vi "Set measurement.vi"(8 "error in (no error)":errorcluster, 10 "Measurement settings":T1={"Source Mode "=0, "Source Level"=0.0, "Source Limit"=0.0, "Measure Function"=1, "Remote sense"=FALSE, "Clear buffer?"=FALSE, "Beep"=FALSE, "High Capacity"=FALSE, "Terminals"=0, "PLCs"=1.0, "Fast measurement"=FALSE} {"Measure Function" items=["Volts", "Current", "Auto Resistance", "Manual Resistance", "Digitize Voltage", "Digitize Current"]; "Source Mode" items=["Voltage", "Current"]; "Terminals" items=["Front", "Rear"]}, 11 "SMU status in":T2 {"Measure Function" items=["Volts", "Current", "Auto Resistance", "Manual Resistance", "Digitize Voltage", "Digitize Current"]; "Source Mode" items=["Voltage", "Current"]}) -> (0 "error out":errorcluster, 3 "SMU status out":T2 {"Measure Function" items=["Volts", "Current", "Auto Resistance", "Manual Resistance", "Digitize Voltage", "Digitize Current"]; "Source Mode" items=["Voltage", "Current"]})   [LabVIEW 2017]
uses:
  ctls/SMU status.ctl
  ctls/SMU settings.ctl
  <instrlib>/Keithley 2450/Keithley 2450.lvlib
  Source meter.lvlib
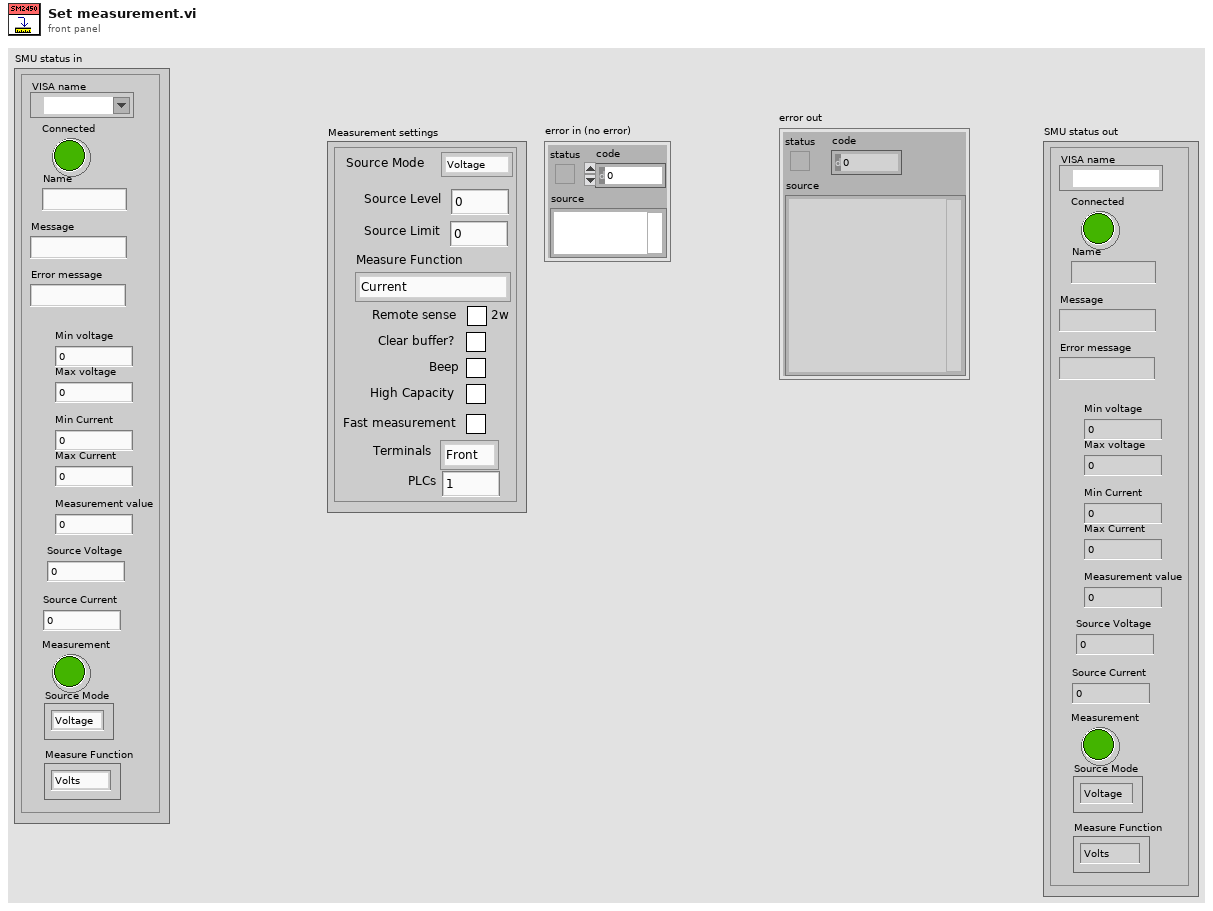
[diagram p1: front panel]
types:
  T1 = typedef "SMU settings.ctl" = cluster{"Source Mode ":u16, "Source Level":dbl, "Source Limit":dbl, "Measure Function":u16, "Remote sense":bool, "Clear buffer?":bool, "Beep":bool, "High Capacity":bool, "Terminals":u16, "PLCs":dbl, "Fast measurement":bool}
  T2 = typedef "Source meter.lvlib/SMU status.ctl" = cluster{"VISA name":refnum<visa-resource-name>, "Connected":bool, "Name":string, "Message":string, "Error message":string, "Min voltage":dbl, "Max voltage":dbl, "Min Current":dbl, "Max Current":dbl, "Measurement value":dbl, "Source Voltage":dbl, "Measurement":bool, "Source Current":dbl, "Source Mode":u16, "Measure Function":u16}
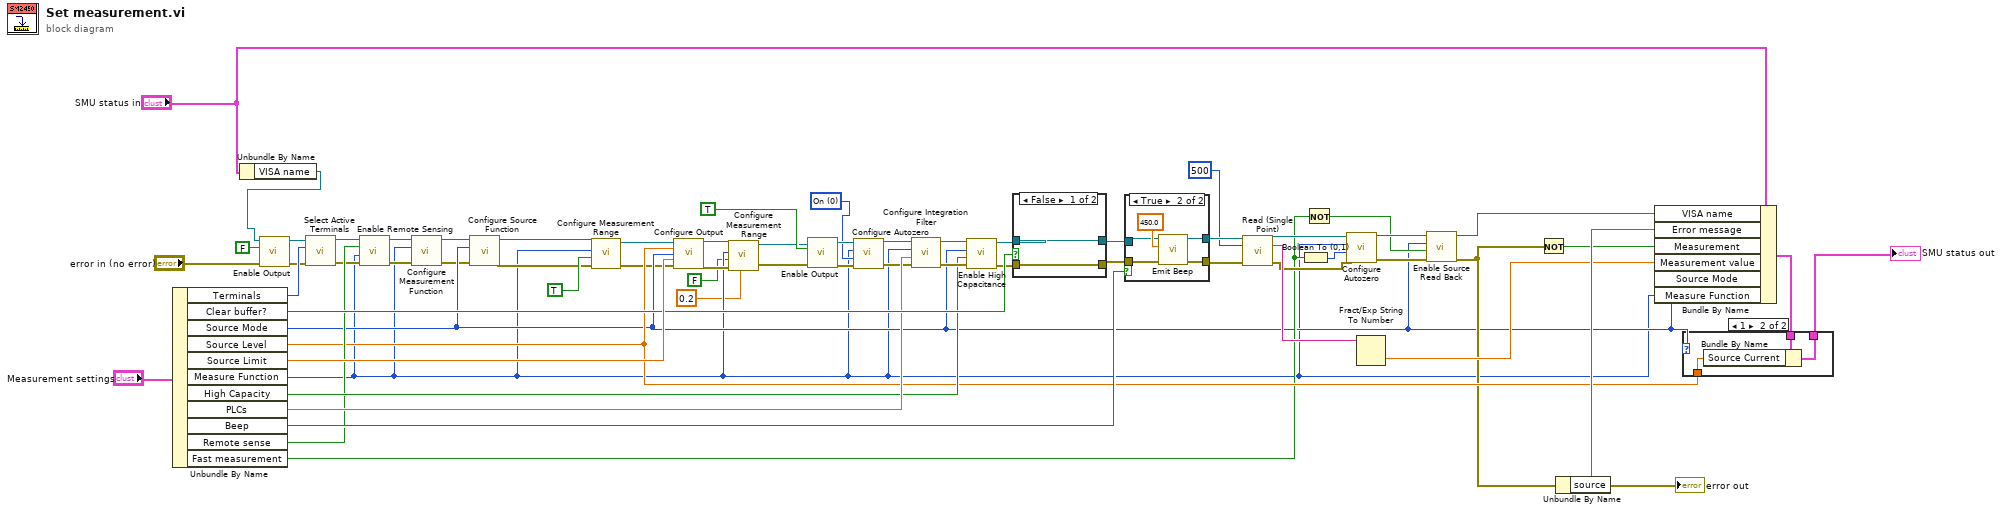
[diagram p0: block diagram]
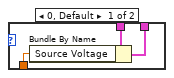
[diagram p2: hidden frame]
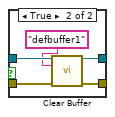
[diagram p4: hidden frame]
diagram:
  w26 = u16 0 items=["On", "Off"] ("Autozero  (0: On)")
  n1 = Unbundle By Name("Measurement settings") -> ("Terminals"=w58:u16, "Clear buffer?"=w54:bool, "Source Mode"=w16:u16, "Source Level"=w34:dbl, "Source Limit"=w57:dbl, "Measure Function"=w3:u16, "High Capacity"=w50:bool, "PLCs"=w53:dbl, "Beep"=w42:bool, "Remote sense"=w41:bool, "Fast measurement"=w23:bool)
  n2 = Unbundle By Name("SMU status in") -> ("VISA name"=w64:refnum<visa-resource-name>)
  n3 = call <instrlib>:"Enable Output.vi"("error in (no error)"="error in (no error)", "Enable Output (T: Enable)"=FALSE, "VISA resource name"=w64) -> ("error out"=w45:errorcluster, "VISA resource name out"=w46:refnum<visa-resource-name>)  [unwired: 7 in]
  n4 = call <instrlib>:"Select Active Terminals.vi"("error in (no error)"=w45, "Active Terminals (0: Front)"=w58, "VISA resource name"=w46) -> ("error out"=w17:errorcluster, "VISA resource name out"=w18:refnum<visa-resource-name>)  [unwired: 7 in]
  n5 = call <instrlib>:"Enable Remote Sensing.vi"("error in (no error)"=w17, "Function (0:Voltage)"=w3, "Enable Remote Sensing (T: Enable)"=w41, "VISA resource name"=w18) -> ("error out"=w13:errorcluster, "VISA resource name out"=w12:refnum<visa-resource-name>)  [unwired: 6 in]
  n6 = call <instrlib>:"Configure Measurement Function.vi"("error in (no error)"=w13, "Function (0: Volts)"=w3, "VISA resource name"=w12) -> ("error out"=w14:errorcluster, "VISA resource name out"=w15:refnum<visa-resource-name>)  [unwired: 7 in]
  n7 = call <instrlib>:"Configure Source Function.vi"("error in (no error)"=w14, "Function (0: Volts)"=w16, "VISA resource name"=w15) -> ("error out"=w9:errorcluster, "VISA resource name out"=w11:refnum<visa-resource-name>)  [unwired: 7 in]
  n8 = call <instrlib>:"Configure Measurement Range.vi"("error in (no error)"=w9, "Enable Auto Range (T:Enable)"=TRUE, "Function (0: Volts)"=w3, "VISA resource name"=w11) -> ("error out"=w10:errorcluster, "VISA resource name out"=w8:refnum<visa-resource-name>)  [unwired: 6 in]
  n9 = call <instrlib>:"Configure Output.vi"("VISA resource name"=w8, "Source Level (0)"=w34, "Source Mode  (0: Voltage)"=w16, "Source Limit Level (0.1)"=w57, "error in (no error)"=w10) -> ("VISA resource name out"=w7:refnum<visa-resource-name>, "error out"=w6:errorcluster)  [unwired: 9 in]
  n10 = call <instrlib>:"Configure Measurement Range.vi"("Manual Range (1.0)"=0.2, "error in (no error)"=w6, "Enable Auto Range (T:Enable)"=FALSE, "Function (0: Volts)"=w3, "VISA resource name"=w7) -> ("error out"=w4:errorcluster, "VISA resource name out"=w5:refnum<visa-resource-name>)  [unwired: 5 in]
  n11 = call <instrlib>:"Enable Output.vi"("error in (no error)"=w4, "Enable Output (T: Enable)"=TRUE ("Enable Remote Sensing (T: Enable)"), "VISA resource name"=w5) -> ("error out"=w27:errorcluster, "VISA resource name out"=w28:refnum<visa-resource-name>)  [unwired: 7 in]
  n12 = call <instrlib>:"Configure Autozero.vi"("error in (no error)"=w27, "Autozero  (0: On)"=w26, "Function (0: Volts)"=w3, "VISA resource name"=w28) -> ("error out"=w29:errorcluster, "VISA resource name out"=w30:refnum<visa-resource-name>)  [unwired: 6 in]
  n13 = call <instrlib>:"Configure Integration Filter.vi"("error in (no error)"=w29, "Measurement Speed (1 PLC)"=w53, "Function (0: Volts)"=w3, "VISA resource name"=w30) -> ("error out"=w52:errorcluster, "VISA resource name out"=w51:refnum<visa-resource-name>)  [unwired: 6 in]
  n14 = call <instrlib>:"Enable High Capacitance.vi"("error in (no error)"=w52, "Enable High Capacitance (T:Enable)"=w50, "Function (0: Volts)"=w16, "VISA resource name"=w51) -> ("error out"=w49:errorcluster, "VISA resource name out"=w48:refnum<visa-resource-name>)  [unwired: 6 in]
  n15 = case shown="False" w54 {
    tunnel: [w66 w71] -> w44
    tunnel: [w65 w70] -> w43
    tunnel: w49 -> [w66 w69]
    tunnel: w48 -> [w65 w68]
    frame False {
    }
    frame True {
      n16 = call <instrlib>:"Clear Buffer.vi"("VISA resource name"=w68, "Buffer Name (defbuffer1)"="defbuffer1", "error in (no error)"=w69) -> ("VISA resource name out"=w70:refnum<visa-resource-name>, "error out"=w71:errorcluster)  [unwired: 11 in]
    }
  }
  n17 = case shown="True" w42 {
    tunnel: [w72 w78] -> w39
    tunnel: [w73 w77] -> w40
    tunnel: w44 -> [w72 w75]
    tunnel: w43 -> [w73 w74]
    frame False {
    }
    frame True {
      n18 = call <instrlib>:"Emit Beep.vi"("error in (no error)"=w75, "Beep Frequency (300)"=450.0, "VISA resource name"=w74) -> ("error out"=w78:errorcluster, "VISA resource name out"=w77:refnum<visa-resource-name>)  [unwired: 7 in]
    }
  }
  n19 = call <instrlib>:"Read (Single Point).vi"("VISA resource name"=w40, "Timeout (10000 ms)"=500, "error in (no error)"=w39) -> ("VISA resource name out"=w32:refnum<visa-resource-name>, "Data out"=w37:string, "error out"=w31:errorcluster)  [unwired: 10 in]
  n20 = Boolean To (0,1)(Boolean=w23) -> (0, 1=w33:i16)
  n21 = Not(x=w23) -> (.not. x?=w22:bool)
  n22 = call <instrlib>:"Configure Autozero.vi"("error in (no error)"=w31, "Autozero  (0: On)"=w33, "Function (0: Volts)"=w3, "VISA resource name"=w32) -> ("error out"=w24:errorcluster, "VISA resource name out"=w25:refnum<visa-resource-name>)  [unwired: 6 in]
  n23 = Fract/Exp String To Number(string=w37) -> (number=w36:dbl)  [unwired: 3 in, 1 out]
  n24 = call <instrlib>:"Enable Source Read Back.vi"("error in (no error)"=w24, "Enable Read Back  (T:Enable)"=w22, "Function (0: Volts)"=w16, "VISA resource name"=w25) -> ("error out"=w20:errorcluster, "VISA resource name out"=w21:refnum<visa-resource-name>)  [unwired: 6 in]
  "error out" <- w20
  n25 = Not(x=w20) -> (.not. x?=w19:bool)
  n26 = Unbundle By Name(w20) -> ("source"=w56:string)
  n27 = Bundle By Name(cluster="SMU status in", "VISA name"=w21, "Error message"=w56, "Measurement"=w19, "Measurement value"=w36, "Source Mode"=w16, "Measure Function"=w3) -> (w62:T2)
  n28 = case shown="1" w16 {
    tunnel: w62 -> [w81 w84]
    tunnel: [w80 w83] -> w35
    tunnel: w34 -> [w79 w82]
    frame 0, Default {
      n29 = Bundle By Name(cluster=w81, "Source Voltage"=w79) -> (w80:T2)
    }
    frame 1 {
      n30 = Bundle By Name(cluster=w84, "Source Current"=w82) -> (w83:T2)
    }
  }
  "SMU status out" <- w35
